vi "Save to Excel file.vi"(7 "sheetname":string="Sheet1", 8 "error in (no error)":errorcluster, 10 "Values":string[][](array[string]), 11 "File Name":path=path "C:/PhaeronGit/LVNPOI/Scratch/test.xls") -> (0 "error out":errorcluster)   [LabVIEW 2013]
doc: "Writes the 2D string array to the named Excel format file."
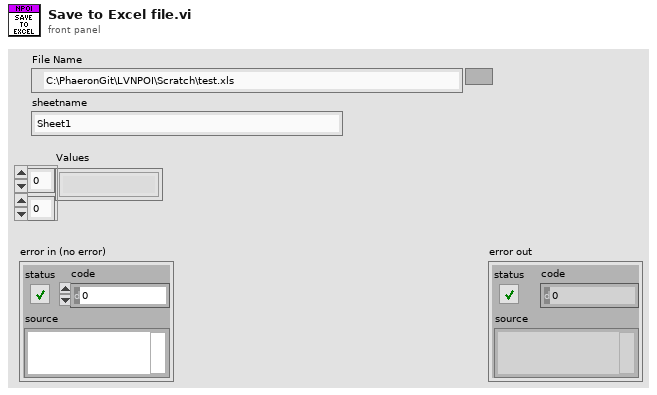
[diagram p1: front panel]
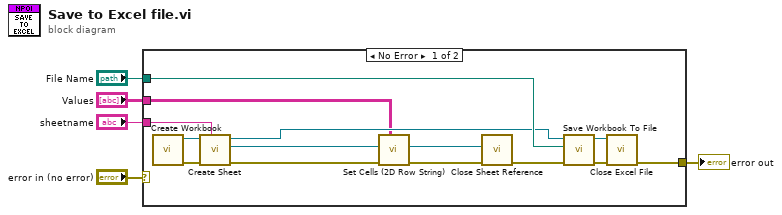
[diagram p0: block diagram]
diagram:
  n1 = case shown="No Error" "error in (no error)" {
    selector: "error in (no error)" -> [_ w20]
    tunnel: "File Name" -> [w19 _]
    tunnel: "sheetname" -> [w18 _]
    tunnel: [w11 w20] -> w3
    tunnel: "Values" -> [w6 _]
    frame No Error {
      n2 = call "Create Workbook.vi"() -> ("error out"=w15:errorcluster, "hssfworkbook"=w16:refnum<k24>)  [unwired: 10 in]
      n3 = call "Create Sheet.vi"("Sheet Name (Sheet1)"=w18, "error in (no error)"=w15, "Workbook Reference"=w16) -> ("error out"=w10:errorcluster, "Sheet Reference"=w8:refnum<k24>, "Workbook Reference"=w17:refnum<k24>)  [unwired: 6 in]
      n4 = call "Set Cells (2D Row String).vi"("Values"=w6, "error in (no error)"=w10, "Sheet Reference"=w8) -> ("error out"=w9:errorcluster, "Sheet Reference out"=w7:refnum<k24>)  [unwired: 7 in]
      n5 = call "Close Sheet Reference.vi"("error in (no error)"=w9, "Sheet Reference"=w7) -> ("error out"=w14:errorcluster)  [unwired: 9 in]
      n6 = call "Save Workbook To File.vi"("error in (no error)"=w14, "File Name"=w19, "Workbook Reference"=w17) -> ("error out"=w13:errorcluster, "Workbook Reference Out"=w12:refnum<k24>)  [unwired: 7 in]
      n7 = call "Close Excel File.vi"("error in (no error)"=w13, "Workbook Reference"=w12) -> ("error out"=w11:errorcluster)  [unwired: 9 in]
    }
    frame Error {
    }
  }
  "error out" <- w3
